vi "STFT vs Time.vi"(0 "scaled signal [EU]":dbl[](array[numeric]) format="%.2f", 1 "window":T3 items=["Rectangle"=0, "Hanning"=1, "Hamming"=2, "Blackman-Harris"=3, "Exact Blackman"=4, "Blackman"=5, "Flat Top"=6, "4 Term B-Harris "=7, "7 Term B-Harris"=8, "Low Sidelobe"=9, "Blackman Nuttall"=11, "Triangle"=30, "Bartlett-Hanning"=31, "Bohman"=32, "Parzen"=33, "Welch"=34, "Kaiser"=60, "Dolph-Chebyshev"=61, "Gaussian"=62], 2 "frequency weighting":T4(ring), 5 "sampling frequency [Hz]":dbl=10000.0 format="%.2f", 7 "time segment":T1={"from [s]"=-1.0, "to [s]"=-1.0, "time increment"=100.0, "time increment units (%)"=enum."%"} {"time increment" format="%.2f"; "to [s]" format="%.2f"; "from [s]" format="%.2f"}, 9 "FFT block size":i32=1024 min=1, 11 "channel info":T2={"sensor sensitivity [mV/EU]"=1000.0, "engineering units"=enum."V", "dB reference [EU]"=1.0, "custom label"="EU", "weighting filter"=enum."Linear", "pregain [dB]"=0.0} {"dB reference [EU]" format="%.1e"; "pregain [dB]" format="%.2f"; "sensor sensitivity [mV/EU]" format="%.2f"}, 12 "dB On (T)":bool=TRUE) -> (4 "power spectrum [EU^2 rms]":dbl[][](array[numeric]) format="%.2f", 6 "unit label":string, 8 "t0 and delta t [s]":cluster{"t0":dbl, "delta t":dbl} {"delta t" format="%.2f"; "t0" format="%.2f"}, 10 "f0 and delta f [Hz]":cluster{"f0":dbl, "delta f":dbl} {"delta f" format="%.2f"; "f0" format="%.2f"}, 15 "weighting conflict":bool)   [LabVIEW 2017]
doc: "Performs an STFT (Short-Time Fourier Transform) on the input signal.\nThe time segment cluster specifies the time segment to analyze and the time increment and its units (%, s, or ms).\nThis VI returns a 2D array that contains the power spectrum at various selected times. The VI also returns the information (t0 and delta t, f0 and delta f) needed to display the results on a colormap or waterfall display."
uses:
  <vilib>/Analysis/4window.llb/windowTd.ctl
  <vilib>/addons/Sound and Vibration/svt_Transients/SoundVib_Transient.lvlib
  <vilib>/Analysis/NI_AALPro.lvlib
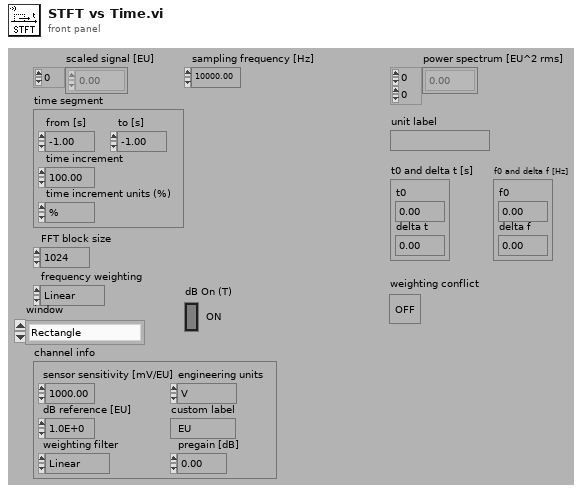
[diagram p1: front panel]
types:
  T1 = cluster{"from [s]":dbl, "to [s]":dbl, "time increment":dbl, "time increment units (%)":enum16{"%", "s", "ms"}}
  T2 = cluster{"sensor sensitivity [mV/EU]":dbl, "engineering units":enum16{"custom...", "V", "Pa", "g", "m/s^2", "m/s", "m", "in/s^2", "in/s", "in"}, "dB reference [EU]":dbl, "custom label":string, "weighting filter":enum16{"Linear", "A-weighting", "B-weighting", "C-weighting"}, "pregain [dB]":dbl}
  T3 = typedef "NI_AALPro.lvlib/windowTd.ctl" = u32
  T4 = enum16{"Linear", "A-weighting", "B-weighting", "C-weighting"}
  T5 = cluster{"FFT block size":i32, "number of FFT":i32, "start index":i32, "increment":dbl}
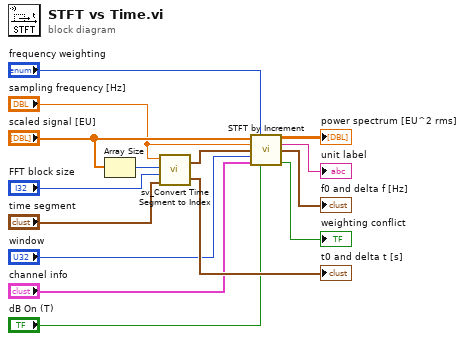
[diagram p0: block diagram]
diagram:
  n1 = Array Size(array="scaled signal [EU]") -> (size(s)=w3:i32)
  n2 = call <vilib>:"sv_Convert Time Segment to Index.vi"("sampling frequency [Hz]"="sampling frequency [Hz]", "array size"=w3, "FFT block size"="FFT block size", "time segment"="time segment") -> ("FFT info"=w12:T5, "to and delta t [s]"=→"t0 and delta t [s]":cluster{"to":dbl, "delta t":dbl})  [unwired: 1 in]
  n3 = call <vilib>:"STFT by Increment.vi"("scaled signal [EU]"="scaled signal [EU]", "frequency weighting"="frequency weighting", "sampling frequency [Hz]"="sampling frequency [Hz]", "FFT info"=w12, "window"="window", "channel info"="channel info", "dB On (T)"="dB On (T)") -> ("power spectrum [EU^2 rms]"=→"power spectrum [EU^2 rms]":dbl[][], "unit label"=→"unit label":string, "f0 and delta f [Hz]"=→"f0 and delta f [Hz]":cluster{"f0":dbl, "delta f":dbl}, "weighting conflict"=→"weighting conflict":bool)  [unwired: 5 in]
